vi "Write Display Metadata.vi"(8 "error in":errorcluster, 10 "Display metadata":T1, 11 "Value in":refnum<class "Value.lvclass">) -> (0 "error out":errorcluster, 3 "Value out":refnum<class "Value.lvclass">)   [LabVIEW 2020, in "Value.lvlib" / "Value.lvclass"]
uses:
  Value.lvclass
  <vilib>/addons/Tools/Unicode/UTF8 Tools.lvlib
  Display Metadata.ctl
  Value.lvlib
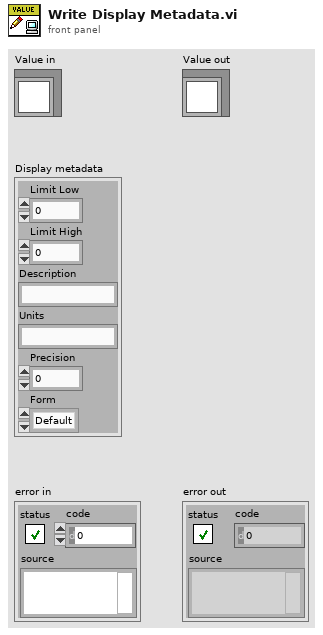
[diagram p1: front panel]
types:
  T1 = typedef "Value.lvlib/Display Metadata.ctl" = cluster{"Limit Low":dbl, "Limit High":dbl, "Description":string, "Units":string, "Precision":i32, "Form":enum32{"Default", "String", "Binary", "Decimal", "Hex", "Exponential", "Engineering"}}
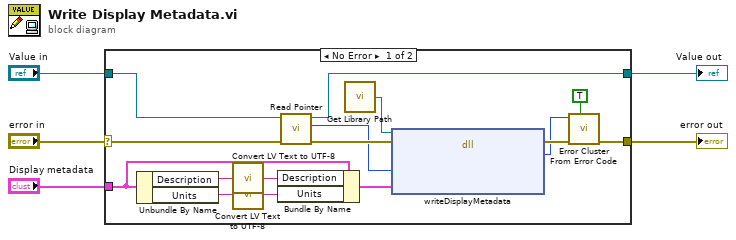
[diagram p0: block diagram]
diagram:
  n1 = case shown="No Error" "error in" {
    selector: "error in" -> [w16 w23]
    tunnel: [w17 w23] -> w5
    tunnel: "Value in" -> [w14 w22]
    tunnel: [w12 w22] -> w2
    tunnel: "Display metadata" -> [w11 _]
    frame No Error {
      n2 = Unbundle By Name(w11) -> ("Description"=w8:string, "Units"=w9:string)
      n3 = call <vilib>:"Convert LV Text to UTF-8.vi"("LV Text"=w8) -> ("UTF-8 Text"=w7:string)  [unwired: 13 in, 1 out]
      n4 = call <vilib>:"Convert LV Text to UTF-8.vi"("LV Text"=w9) -> ("UTF-8 Text"=w6:string)  [unwired: 13 in, 1 out]
      n5 = Bundle By Name(cluster=w11, "Description"=w7, "Units"=w6) -> (w10:T1)
      n6 = call-dynamic "Read Pointer.vi"("error in (no error)"=w16, "Value in"=w14) -> ("error out"=w15:errorcluster, "pointer"=w13:i64, "Value out"=w12:refnum<class "Value.lvclass">)  [unwired: 7 in]
      n7 = call "Get Library Path.vi"() -> ("Path"=w21:path)  [unwired: 1 in]
      n8 = dll-call lib="?" fn="writeDisplayMetadata"(path in=w21, error in=w15, "value"=w13, "display metadata"=w10) -> (error out=w19:errorcluster, "err_code"=w18:i32)  [unwired: 3 in, 1 out]
      n9 = call <vilib>:"Error Cluster From Error Code.vi"("show call chain? (False)"=TRUE, "error in (no error)"=w19, "error code (0)"=w18) -> ("error out"=w17:errorcluster)  [unwired: 6 in]
    }
    frame Error {
    }
  }
  "error out" <- w5
  "Value out" <- w2
